vi "Channel1.vi"(4 "Physical Channel 9":tag="Dev1/ai1", 6 "Maximum Value 9":dbl=2.0 format="%0.3f", 7 "avg num 5":i32=10, 10 "Minimum Value 9":dbl=-2.0 format="%0.3f", 11 "?":bool) -> (2 "Array":dbl[](array[numeric]), 3 "pH voltage 3":dbl(graph)=1.4077970382798781)   [LabVIEW 2018]
uses:
  <vilib>/Utility/error.llb/DialogType.ctl
  <vilib>/DAQmx/read.llb/DAQmx Read (Analog DBL 1Chan 1Samp).vi
  <vilib>/DAQmx/create/channels.llb/DAQmx Create Channel (AI-Voltage-Basic).vi
  <vilib>/DAQmx/miscellaneous.llb/DAQmx Fill In Error Info.vi
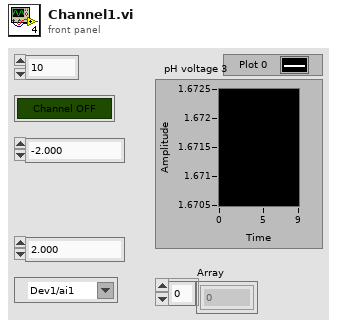
[diagram p1: front panel]
types:
  T1 = typedef "DialogType.ctl" = u16
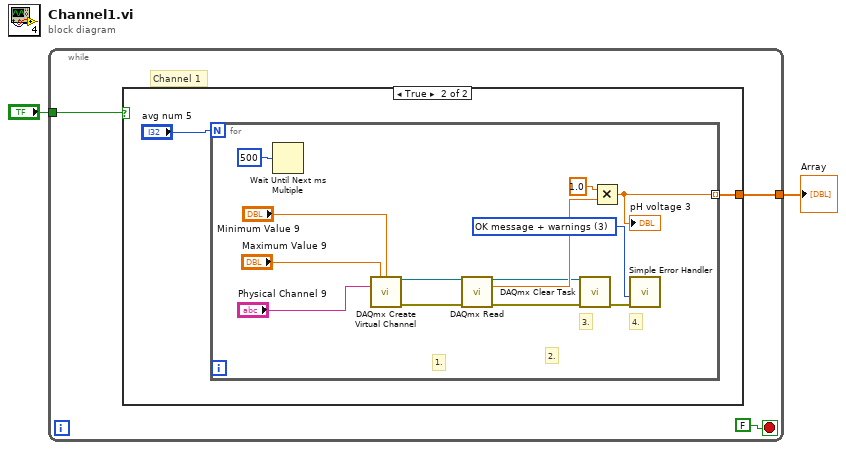
[diagram p0: block diagram]
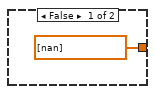
[diagram p2: hidden frame]
diagram:
  n1 = while {
    tunnel: [w5] -> w2
    tunnel: "?" -> [w3]
    stop <- FALSE stop-if-true
    # "Channel 1"
    n2 = case shown="True" w3 {
      tunnel: [dbl[] [nan] w8] -> w5
      frame False {
      }
      frame True {
        n3 = for {
          N: "avg num 5" -> [_]
          tunnel: [w11] -> w8 mode=indexing
          w16 = T1 3 items=["no dialog", "OK message", "continue or stop message", "OK message + warnings", "continue/stop + warnings"] ("type of dialog (OK msg:1)")
          # "3."
          # "2."
          # "4."
          # "1."
          n4 = Wait Until Next ms Multiple(millisecond multiple=u32 500) -> ()  [unwired: 1 out]
          n5 = call-poly <vilib>:"DAQmx Create Virtual Channel.vi"("maximum value"="Maximum Value 9", "minimum value"="Minimum Value 9", "physical channels"="Physical Channel 9") -> ("task out"=w10:refnum<k21>, "error out"=w9:errorcluster)  [unwired: 11 in]
          n6 = call-poly <vilib>:"DAQmx Read.vi"("task/channels in"=w10, "error in"=w9) -> ("task out"=w17:refnum<k21>, "data"=w21:dbl, "error out"=w18:errorcluster)  [unwired: 11 in]
          n7 = call <vilib>:"DAQmx Clear Task.vi"("task in"=w17, "error in"=w18) -> ("error out"=w19:errorcluster)  [unwired: 13 in]
          n8 = Multiply(x=1.0, y=w21) -> (x*y=w11:dbl)
          "pH voltage 3" <- w11
          n9 = call <vilib>:"Simple Error Handler.vi"("type of dialog (OK msg:1)"=w16, "error in (no error)"=w19) -> ()  [unwired: 3 in, 5 out]
        }
      }
    }
  }
  "Array" <- w2
